vi "KalmanFilter_GetXHat_Single.vi"(9 "Row":i32, 11 "in KalmanFilter":T1) -> (3 "xHat":dbl)   [LabVIEW 2019, in "Trajectory_Library.lvlib"]
doc: "Returns a single element of the state estimate x-hat.\n \nInputs:\n - KalmanFilter -- filter data cluster\n - row -- matrix row number (0-n)\n\nOutputs:\n - xHat - The single state estimate x-hat value."
uses:
  Trajectory_Library.lvlib
  TypeDef/KALMAN_FILTER.ctl
  <vilib>/Analysis/Matrix/Datatypes/RealMatrix.ctl
  TypeDef/LINEAR_SYSTEM.ctl
  <vilib>/Analysis/Matrix/NI_Matrix.lvlib
panel:
  # "Steady State Gain  \n<States,Outputs>"
  # "State Estimate <Statess,1>"
  # "<States,States>"
  # "<States,Inputs>"
  # "<Outputs,States>"
  # "<Outputs,Inputs>"
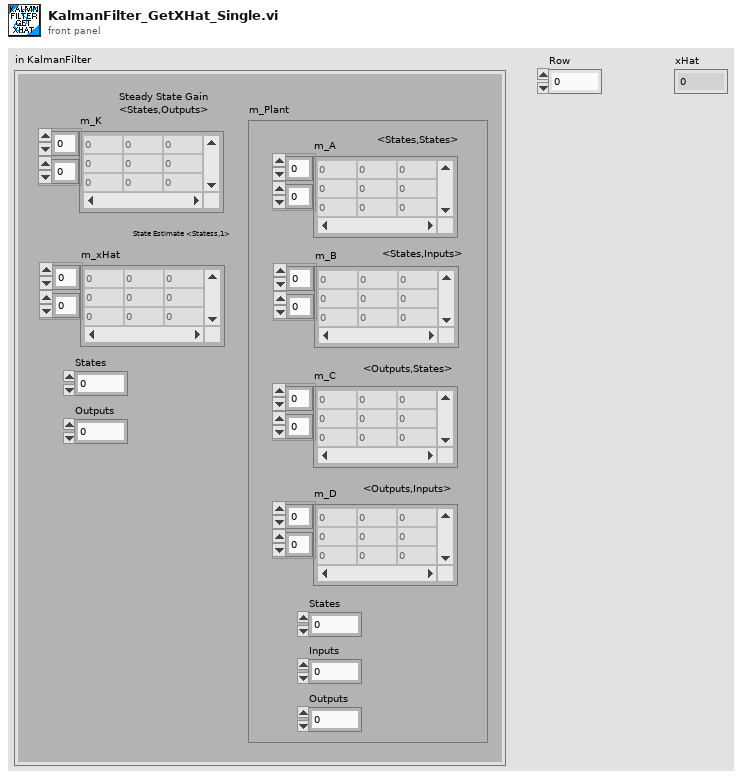
[diagram p1: front panel]
types:
  T1 = typedef "Trajectory_Library.lvlib/KALMAN_FILTER.ctl" = cluster{"m_K":T2, "m_xHat":T2, "States":i32, "Outputs":i32, "m_Plant":T3}
  T2 = typedef "NI_Matrix.lvlib/RealMatrix.ctl" = dbl[][]
  T3 = typedef "Trajectory_Library.lvlib/LINEAR_SYSTEM.ctl" = cluster{"m_A":T2, "m_B":T2, "m_C":T2, "m_D":T2, "States":i32, "Inputs":i32, "Outputs":i32}
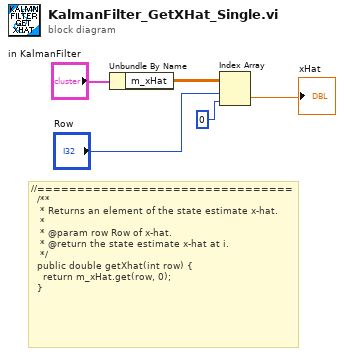
[diagram p0: block diagram]
diagram:
  # "//================================\n  /**\n   * Returns an element of the state estimate x-hat.\n   *\n   * @param row Row of x-hat.\n   * @return the state estimate x-hat at i.\n   */\n  public double getXhat(int row) {\n    return m_xHat.get(row, 0);\n  }"
  n1 = Unbundle By Name("in KalmanFilter") -> ("m_xHat"=w4:T2)
  n2 = Index Array(array=w4, index (row)="Row", index (col)=0) -> (element=→"xHat":dbl)
